vi "Read Graph Data.vi"() -> ()   [LabVIEW 2020]
uses:
  _libraries/Startup Processes/_typedefs/Subpanel Names.ctl
  toolbox/Standard Signalling/not_Generic Named Notifier/not_Generic Named Notifier.lvlib
  _ude/Read Graph Data/Read Graph Data.lvlib
  _libraries/Startup Processes/Startup Processes.lvlib
panel:
  out "Raw Response":variant
  out "Waveform Graph":dbl[](graph)
  out "Error Out":errorcluster
  in  "Plugin Names":T1
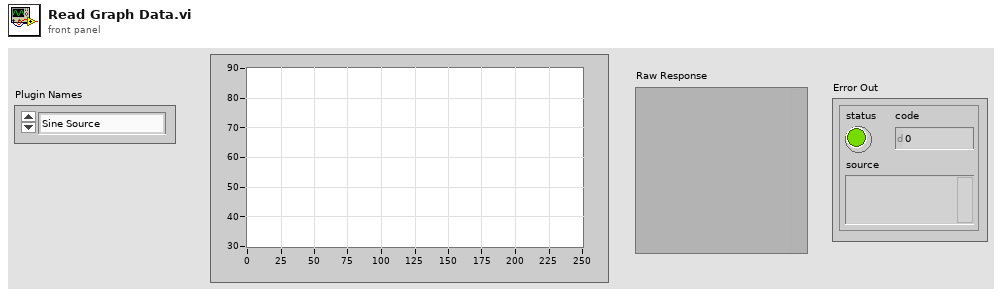
[diagram p1: front panel]
types:
  T1 = typedef "Startup Processes.lvlib/Subpanel Names.ctl" = enum16{"Sine Source", "Ramp Source", "Hen House TC", "Dog House TC", "Out House TC"}
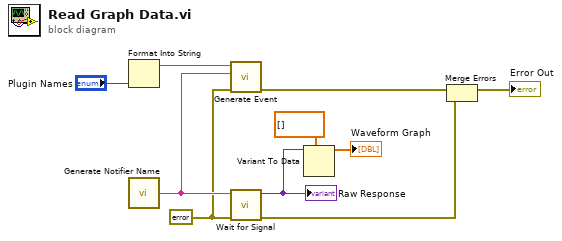
[diagram p0: block diagram]
diagram:
  w5 = errorcluster {"status"=FALSE, "code"=0, "source"=""} ("Error In")
  n1 = Format Into String("Plugin Names") -> (resulting string=w7:string)  [unwired: 3 in, 1 out]
  n2 = call "Generate Notifier Name.vi"() -> ("Notifier Name"=w6:string)
  n3 = call "Generate Event.vi"("Error In"=w5, "Response Notifier"=w6, "Graph Name"=w7) -> ("Error Out"=w4:errorcluster)  [unwired: 4 in]
  n4 = call "Wait for Signal.vi"("Error In"=w5, "Notifier Name"=w6) -> ("Error Out"=w8:errorcluster, "Signal Data"=w1:variant)  [unwired: 4 in]
  "Raw Response" <- w1
  n5 = Variant To Data(type=dbl[] [] ("Waveform Graph"), Variant=w1) -> (data=→"Waveform Graph":dbl[])  [unwired: 1 in, 1 out]
  n6 = Merge Errors(w4, w8) -> (→"Error Out":errorcluster)
